vi "RandomArray_D.vi"(9 "N":dbl=1.0 min=1.0, 10 "Min":dbl, 11 "Max 2":dbl=1.0) -> (3 "Array":dbl[](array[numeric]))   [LabVIEW 2013]
panel:
  out "Waveform Graph":dbl[](graph)
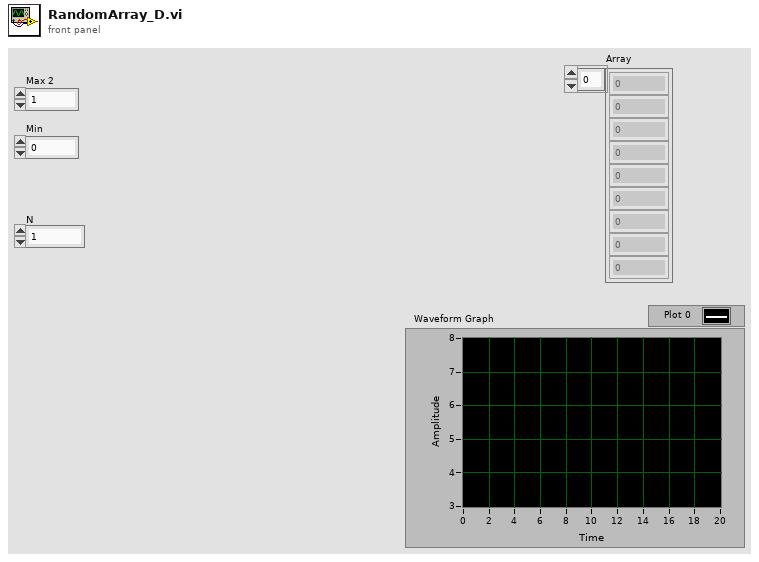
[diagram p1: front panel]
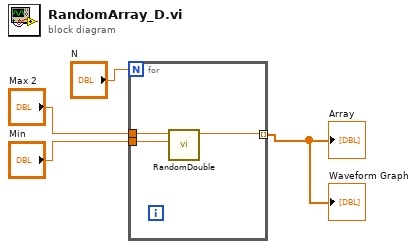
[diagram p0: block diagram]
diagram:
  n1 = for {
    N: "N" -> [_]
    tunnel: "Max 2" -> [w7]
    tunnel: "Min" -> [w6]
    tunnel: [w5] -> w1 mode=indexing
    n2 = call "RandomDouble.vi"("Min"=w6, "Max"=w7) -> ("Random"=w5:dbl)  [unwired: 9 in]
  }
  "Array" <- w1
  "Waveform Graph" <- w1
